vi "Scan Setup.vi"(8 "error in (no error)":errorcluster, 11 "PC Reader in":refnum<class "Photon Counter Reader.lvclass">) -> (0 "error out":errorcluster, 3 "PC Reader out":refnum<class "Photon Counter Reader.lvclass">)   [LabVIEW 2017, in "Photon Counter Reader.lvclass"]
doc: "(Dynamic) Send commands to configure the instrument based on the class member data."
uses:
  Photon Counter Reader.lvclass
  Photon Counter Reader.lvclass/Photon Counter Reader.ctl
  Reader/Reader.lvclass
  Instruments/Utility Classes/Readable/Readable.lvclass
  Instruments/Photon Counter/SR400/SR400.lvlib
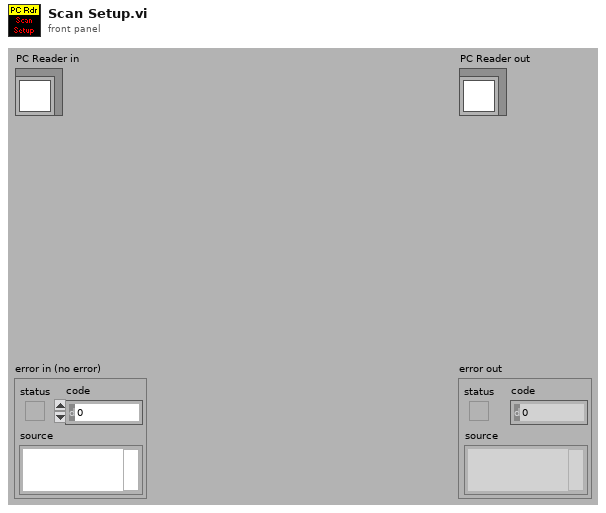
[diagram p1: front panel]
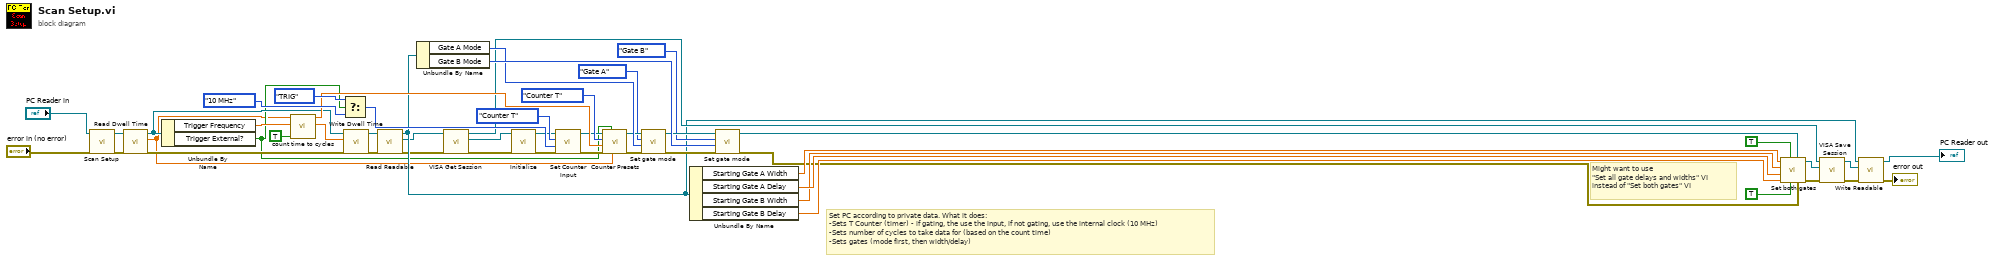
[diagram p0: block diagram]
diagram:
  # "Might want to use \n\"Set all gate delays and widths\" VI \ninstead of \"Set both gates\" VI"
  # "Set PC according to private data. What it does:\n-Sets T Counter (timer) - if gating, the use the input, if not gating, use the internal clock (10 MHz)\n-Sets number of cycles to take data for (based on the count time)\n-Sets gates (mode first, then width/delay)"
  n1 = call-parent "Scan Setup.vi"("error in (no error)"="error in (no error)", "Reader in"="PC Reader in") -> ("error out"=w15:errorcluster, "Reader out"=w17:refnum<class "Photon Counter Reader.lvclass">)  [unwired: 8 out]
  n2 = call-dynamic "Read Dwell Time.vi"("error in (no error)"=w15, "Reader.lvclass in"=w17) -> ("error out"=w13:errorcluster, "Dwell Time"=w1:dbl[unit], "Reader.lvclass out"=w16:refnum<class "Photon Counter Reader.lvclass">)  [unwired: 7 out]
  n3 = Unbundle By Name(w16) -> ("Trigger Frequency"=w28:dbl[unit], "Trigger External?"=w2:bool)
  n4 = call "count time to cycles.vi"("dispmsg?"=TRUE, "Trigger Freq"=w28, "Count Time Set"=w1) -> ("Count Time Current"=w14:dbl[unit], "Number of triggers"=w27:dbl)  [unwired: 3 out]
  n5 = Select(t=enum16{"10 MHz", "INPUT 1", "INPUT 2", "TRIG"}."TRIG" ("Input (def: 10 MHz)"), s=w2, f=enum16{"10 MHz", "INPUT 1", "INPUT 2", "TRIG"}."10 MHz" ("Input (def: 10 MHz)")) -> (s? t:f=w31:enum16{"10 MHz", "INPUT 1", "INPUT 2", "TRIG"})
  n6 = call-dynamic "Write Dwell Time.vi"("error in (no error)"=w13, "Dwell Time"=w14, "Reader.lvclass in"=w16) -> ("error out"=w5:errorcluster, "Reader.lvclass out"=w12:refnum<class "Photon Counter Reader.lvclass">)  [unwired: 7 out]
  n7 = call-dynamic "Read Readable.vi"("error in (no error)"=w5, "Reader.lvclass in"=w12) -> ("error out"=w6:errorcluster, "Readable.lvclass"=w4:refnum<class "Readable.lvclass">, "Reader.lvclass out"=w11:refnum<class "Photon Counter Reader.lvclass">)  [unwired: 7 out]
  n8 = Unbundle By Name(w11) -> ("Gate A Mode"=w41:u16, "Gate B Mode"=w42:u16)
  n9 = call-dynamic "VISA Get Session.vi"("error in (no error)"=w6, "Instrument.lvclass in"=w4) -> ("error out"=w7:errorcluster, "VISA Resource Name"=w10:refnum<visa-resource-name>, "Instrument.lvclass out"=w21:refnum<class "Readable.lvclass">)  [unwired: 7 out]
  n10 = call "Initialize.vi"("errorIN"=w7, "VISA resource name"=w10) -> ("errorOUT"=w8:errorcluster, "VISA resource name out"=w9:refnum<visa-resource-name>)  [unwired: 8 out]
  n11 = call "Set Counter Input.vi"("error in (no error)"=w8, "Input (def: 10 MHz)"=w31, "Counter (def: A)"=enum16{"Counter A", "Counter B", "Counter T"}."Counter T" ("i (0) 2"), "VISA resource name"=w9) -> ("error out"=w23:errorcluster, "VISA resource name out"=w22:refnum<visa-resource-name>)  [unwired: 6 out]
  n12 = call "Counter Presets.vi"("T_set"=w1, "Trigger external?"=w2, "error in (no error)"=w23, "Number of triggers"=w27, "Counter (Def: T)"=enum16{"Invalid", "Counter B", "Counter T"}."Counter T" ("i (0) 2"), "VISA resource name"=w22) -> ("error out"=w34:errorcluster, "VISA resource name out"=w37:refnum<visa-resource-name>)  [unwired: 4 out]
  n13 = call "Set gate mode.vi"("error in (no error)"=w34, "Mode (def: CW)"=w41, "Gate (def: A)"=enum16{"Gate A", "Gate B"}."Gate A", "VISA resource name"=w37) -> ("error out"=w35:errorcluster, "VISA resource name out"=w36:refnum<visa-resource-name>)  [unwired: 6 out]
  n14 = Unbundle By Name(w11) -> ("Starting Gate A Width"=w43:dbl[unit], "Starting Gate A Delay"=w45:dbl[unit], "Starting Gate B Width"=w44:dbl[unit], "Starting Gate B Delay"=w46:dbl[unit])
  n15 = call "Set gate mode.vi"("error in (no error)"=w35, "Mode (def: CW)"=w42, "Gate (def: A)"=enum16{"Gate A", "Gate B"}."Gate B", "VISA resource name"=w36) -> ("error out"=w39:errorcluster, "VISA resource name out"=w38:refnum<visa-resource-name>)  [unwired: 6 out]
  n16 = call "Set both gates.vi"("Error In"=w39, "VISA resource name"=w38, "Set Delay?"=TRUE, "Set Width?"=TRUE, "gatedelayoffsetB"=w46, "gatedelayoffsetA"=w45, "Gate B Width"=w44, "Gate A Width"=w43) -> ("Error Out"=w40:errorcluster, "VISA resource name out"=w49:refnum<visa-resource-name>)  [unwired: 2 out]
  n17 = call-dynamic "VISA Save Session.vi"("error in (no error)"=w40, "VISA Resource Name"=w49, "Instrument.lvclass in"=w21) -> ("error out"=w19:errorcluster, "Instrument.lvclass out"=w20:refnum<class "Readable.lvclass">)  [unwired: 7 out]
  n18 = call-dynamic "Write Readable.vi"("error in (no error)"=w19, "Readable.lvclass"=w20, "Reader.lvclass in"=w11) -> ("error out"=→"error out":errorcluster, "Reader.lvclass out"=→"PC Reader out":refnum<class "Photon Counter Reader.lvclass">)  [unwired: 7 out]
